vi "ex14-4.vi"() -> ()   [LabVIEW 2014]
uses:
  <vilib>/NXT/Subs/MotorOutput.ctl
  <vilib>/NXT/Dual Mode Library/Motors/MotorDistance_Single.vi
  <vilib>/NXT/Dual Mode Library/Display/drawNumber.vi
panel:
  out "二進位顯示":dbl[](array[numeric])
  out "紙帶所代表數值":i32
  in  "光值判斷":i16
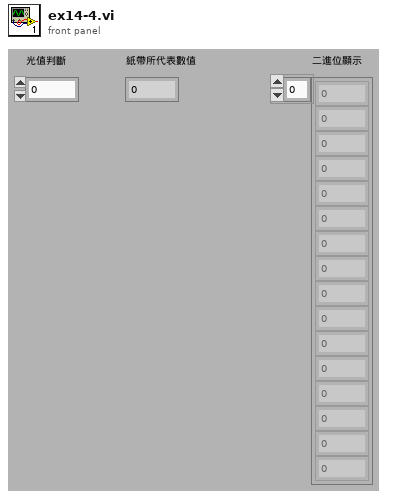
[diagram p1: front panel]
types:
  T1 = typedef "MotorOutput.ctl" = u8
  T2 = typedef "LVHSConnector.ctl" = refnum<class "BrickReference.lvclass">
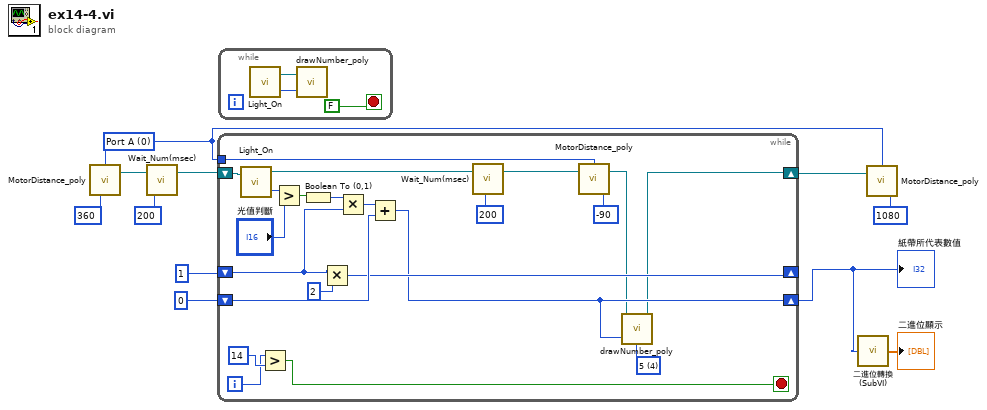
[diagram p0: block diagram]
diagram:
  w8 = T1 0 items=["Port A", "Port B", "Port C", "All Ports"] ("Output Port (All Ports)")
  n1 = call-poly <vilib>:"MotorDistance_poly.vi"("Angle of Rotation (360)"=360 ("Distance (100)"), "Output Port (All Ports)"=w8) -> ("NXT/EV3"=w5:T2)  [unwired: 2 in]
  n2 = call <vilib>:"Wait_Num(msec).vi"("Time (100 msec)"=u32 200, "NXT/EV3"=w5) -> ("NXT/EV3"=w4:T2)  [unwired: 2 in]
  n3 = while {
    shift-right: [w25] -> _
    shift-left: 1 -> [w27]
    shift-right: [w16] -> w1
    shift-left: 0 -> [w28]
    tunnel: w8 -> [w24]
    shift-right: [w13] -> w6
    shift-left: w4 -> [w21]
    i -> [w19]
    stop <- w22 stop-if-true
    w15 = i16 4 items=["1", "2", "3", "4", "5", "6", "7", "8"] ("Line")
    n4 = call <vilib>:"Light_On.vi"("NXT/EV3"=w21) -> ("Scaled Value"=w33:i16, "NXT/EV3"=w17:T2)  [unwired: 2 in]
    n5 = Greater?(x=w19, y=14 ("x")) -> (0:w22:bool)
    n6 = Greater?(x=w33, y="光值判斷") -> (0:w31:bool)
    n7 = Boolean To (0,1)(Boolean=w31) -> (0, 1=w30:i16)
    n8 = Multiply(x=w27, y=2) -> (x*y=w25:i32)
    n9 = Multiply(x=w30, y=w27) -> (x*y=w29:i32)
    n10 = Add(x=w29, y=w28) -> (x+y=w16:i32)
    n11 = call <vilib>:"Wait_Num(msec).vi"("Time (100 msec)"=u32 200, "NXT/EV3"=w17) -> ("NXT/EV3"=w18:T2)  [unwired: 2 in]
    n12 = call-poly <vilib>:"MotorDistance_poly.vi"("Angle of Rotation (360)"=-90 ("Distance (100)"), "NXT/EV3"=w18, "Output Port (All Ports)"=w24) -> ("NXT/EV3"=w14:T2)  [unwired: 1 in]
    n13 = call-poly <vilib>:"drawNumber_poly.vi"("number"=w16, "NXT/EV3"=w14, "Line"=w15) -> ("NXT/EV3"=w13:T2)  [unwired: 1 in]
  }
  "紙帶所代表數值" <- w1
  n14 = while {
    stop <- FALSE stop-if-true
    n15 = call <vilib>:"Light_On.vi"() -> ("Scaled Value"=w36:i16, "NXT/EV3"=w35:T2)  [unwired: 3 in]
    n16 = call-poly <vilib>:"drawNumber_poly.vi"("number"=w36, "NXT/EV3"=w35) -> ()  [unwired: 2 in, 1 out]
  }
  n17 = call "二進位轉換 (SubVI).vi"("十進位"=w1) -> ("二進位"=→"二進位顯示":dbl[])
  n18 = call-poly <vilib>:"MotorDistance_poly.vi"("Angle of Rotation (360)"=1080 ("Distance (100)"), "NXT/EV3"=w6, "Output Port (All Ports)"=w8) -> ()  [unwired: 1 in, 1 out]
